vi "Begin.vi"(10 "Control Type":i8, 11 "Image Size":T1=enum."160x120") -> (0 "error out":errorcluster)   [LabVIEW 2011]
doc: "Called before other user functions, this VI is expected to open initial I/O refnums, load in file data, and do all program initialization. Notice that the <B>error out</B> terminal is simply used for data flow. Wiring it to other structures or subVIs ensures that this VI runs first."
uses:
  <vilib>/Rock Robotics/WPI/Camera/WPI_CameraImageSize.ctl
  <vilib>/Rock Robotics/WPI/Camera/WPI_CameraWhite Balance Values.ctl
  <vilib>/Rock Robotics/WPI/Camera/WPI_CameraExposure Values.ctl
  <vilib>/Rock Robotics/WPI/Camera/WPI_CameraFrameRate.ctl
  <vilib>/Rock Robotics/SystemInterfaces/Typedef/FPGA_TypedefAnalogModuleForGyro.ctl
  <vilib>/Rock Robotics/SystemInterfaces/AI/FPGA_AIGyroChannel.ctl
  <vilib>/Rock Robotics/SystemInterfaces/DIO/FPGA_DIOPWMChannel.ctl
  <vilib>/Rock Robotics/SystemInterfaces/Typedef/FPGA_TypedefDigitalModule.ctl
  <vilib>/Rock Robotics/SystemInterfaces/DIO/FPGA_DIOChannel.ctl
  <vilib>/Rock Robotics/SystemInterfaces/Typedef/FPGA_TypedefAnalogModule.ctl
  <vilib>/Rock Robotics/SystemInterfaces/AI/FPGA_AIChannel.ctl
  <vilib>/Rock Robotics/WPI/Encoder/WPI_EncoderType.ctl
  <vilib>/Rock Robotics/WPI/Joystick/WPI_JoystickDeviceEnum.ctl
  <vilib>/Rock Robotics/WPI/MotorControl/WPI_MotorControlOpen Victor.vi
  <vilib>/Rock Robotics/WPI/Counter/WPI_CounterDigitalInputToDigitalSource.vi
  <vilib>/Rock Robotics/WPI/RobotDrive/WPI_RobotDriveOpen4MotorWithVictor.vi
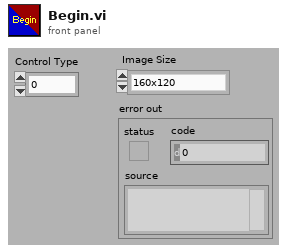
[diagram p1: front panel]
types:
  T1 = typedef "WPI_CameraImageSize.ctl" = enum16{"640x480", "320x240", "160x120"}
  T2 = typedef "WPI_EncoderType.ctl" = enum16{"1x", "2x", "4x"}
  T3 = typedef "FPGA_DIOChannel.ctl" = enum8{"DIO 1", "DIO 2", "DIO 3", "DIO 4", "DIO 5", "DIO 6", "DIO 7", "DIO 8", "DIO 9", "DIO 10", "DIO 11", "DIO 12", "DIO 13", "DIO 14", "Invalid"}
  T4 = typedef "FPGA_TypedefDigitalModule.ctl" = enum16{"Digital Module 1", "Digital Module 2"}
  T5 = typedef "FPGA_AIChannel.ctl" = enum8{"AI 1", "AI 2", "AI 3", "AI 4", "AI 5", "AI 6", "AI 7", "AI 8", "Invalid"}
  T6 = typedef "FPGA_TypedefAnalogModule.ctl" = enum16{"Analog Module 1", "Analog Module 2"}
  T7 = typedef "FPGA_DIOPWMChannel.ctl" = enum8{"PWM 1", "PWM 2", "PWM 3", "PWM 4", "PWM 5", "PWM 6", "PWM 7", "PWM 8", "PWM 9", "PWM 10", "Invalid"}
  T8 = typedef "FPGA_AIGyroChannel.ctl" = enum8{"AI 1", "AI 2", "Invalid"}
  T9 = typedef "FPGA_TypedefAnalogModuleForGyro.ctl" = enum16{"Analog Module 1"}
  T10 = typedef "WPI_CameraFrameRate.ctl" = u32
  T11 = typedef "WPI_CameraExposure Values.ctl" = enum16{"Auto", "Flicker-free 50 Hz", "Flicker-free 60 Hz", "Hold current"}
  T12 = typedef "WPI_CameraWhite Balance Values.ctl" = enum16{"Auto", "Fixed indoor", "Fixed outdoor 1", "Fixed outdoor 2", "Fixed fluorescent 1", "Fixed fluorescent 2", "Hold current"}
  T13 = typedef "WPI_MotorControlDeviceRef.ctl" = cluster{"DeviceStatus":errorcluster, "Type":enum16{"PWM", "CAN"}, "PWM":cluster{"Digital Module":T4, "PWM Channel":T7, "DeadBand":T14}, "CAN":cluster{"Device Number":u8, "Control Mode":T15, "Semaphore":T16, "Max Vout":dbl}, "Invert":bool, "TransformRef":T17, "InvTransformRef":T17}
  T14 = typedef "WPI_PWMDeadband.ctl" = cluster{"Name":string, "maxPositivePwm":i32, "minPositivePwm":i32, "centerPwm":i32, "maxNegativePwm":i32, "minNegativePwm":i32, "angularRange":u16}
  T15 = typedef "WPI_CANJaguar_ControlMode.ctl" = enum8{"Percent VBus", "Current", "Speed", "Position", "Voltage"}
  T16 = typedef "Semaphore RefNum" = refnum<k1>
  T17 = typedef "WPI_PWMTransform_ConPane.ctl" = refnum<vi>
  T18 = typedef "WPI_CameraDevRef.ctl" = cluster{"Camera Address":string, "CameraStatus":errorcluster, "Acquire Image Notifier":refnum<notifier>}
  T19 = typedef "WPI_RobotDriveDevRef.ctl" = cluster{"DevStatus":errorcluster, "Motors[]":T13[], "Square Inputs":bool, "Max Output":dbl, "Isochronous":bool}
  T20 = typedef "WPI_DigitalInputDevRef.ctl" = cluster{"DevStatus":errorcluster, "DIO Channel":T3, "Digital Module":T4}
  T21 = typedef "WPI_AnalogChannelDevRef.ctl" = cluster{"DevStatus":errorcluster, "Analog Module":T6, "Analog Channel":T5}
  T22 = typedef "WPI_GyroDevRef.ctl" = cluster{"DevStatus":errorcluster, "Analog Module":T6, "Analog Channel":T5, "Offset":dbl, "Gain (VoltsPerDegree/Second)":dbl}
  T23 = typedef "FPGA_CounterEncoderSourceConvertionLVSourceType.ctl" = cluster{"DevStatus":errorcluster, "AnalogTriggerMode?":bool, "DigitalMode":cluster{"Digital Module":T4, "DIO Channel":T24}, "AnalogTriggerMode":cluster{"AnalogTriggerIndex":T25, "OutputType":T26}}
  T24 = typedef "FPGA_DIODigitalSourceChannel.ctl" = enum8{"DIO 1", "DIO 2", "DIO 3", "DIO 4", "DIO 5", "DIO 6", "DIO 7", "DIO 8", "DIO 9", "DIO 10", "DIO 11", "DIO 12", "DIO 13", "DIO 14", "Disabled"}
  T25 = typedef "FPGA_AnalogTriggerIndex.ctl" = enum8{"Trig 0", "Trig 1", "Trig 2", "Trig 3", "Trig 4", "Trig 5", "Trig 6", "Trig 7", "Invalid"}
  T26 = typedef "FPGA_AnalogTriggerOutType.ctl" = enum16{"InWindow", "TriggerState", "Rising", "Falling"}
  T27 = typedef "WPI_EncoderDevRef.ctl" = cluster{"DevStatus":errorcluster, "EncoderIndex":T28, "CounterIndex":T29, "DistancePerCount":dbl, "Decoding Type":T2}
  T28 = typedef "FPGA_EncoderIdx.ctl" = enum8{"Enc 0", "Enc 1", "Enc 2", "Enc 3", "Invalid"}
  T29 = typedef "FPGA_CounterCtrSystemIndex.ctl" = enum8{"Ctr 0", "Ctr 1", "Ctr 2", "Ctr 3", "Ctr 4", "Ctr 5", "Ctr 6", "Ctr 7", "Invalid"}
  T30 = typedef "WPI_JoystickDeviceEnum.ctl" = enum16{"USB 1", "USB 2", "USB 3", "USB 4", "Kinect 1", "Kinect 2"}
  T31 = typedef "WPI_JoystickDevRef.ctl" = cluster{"Device":T30}
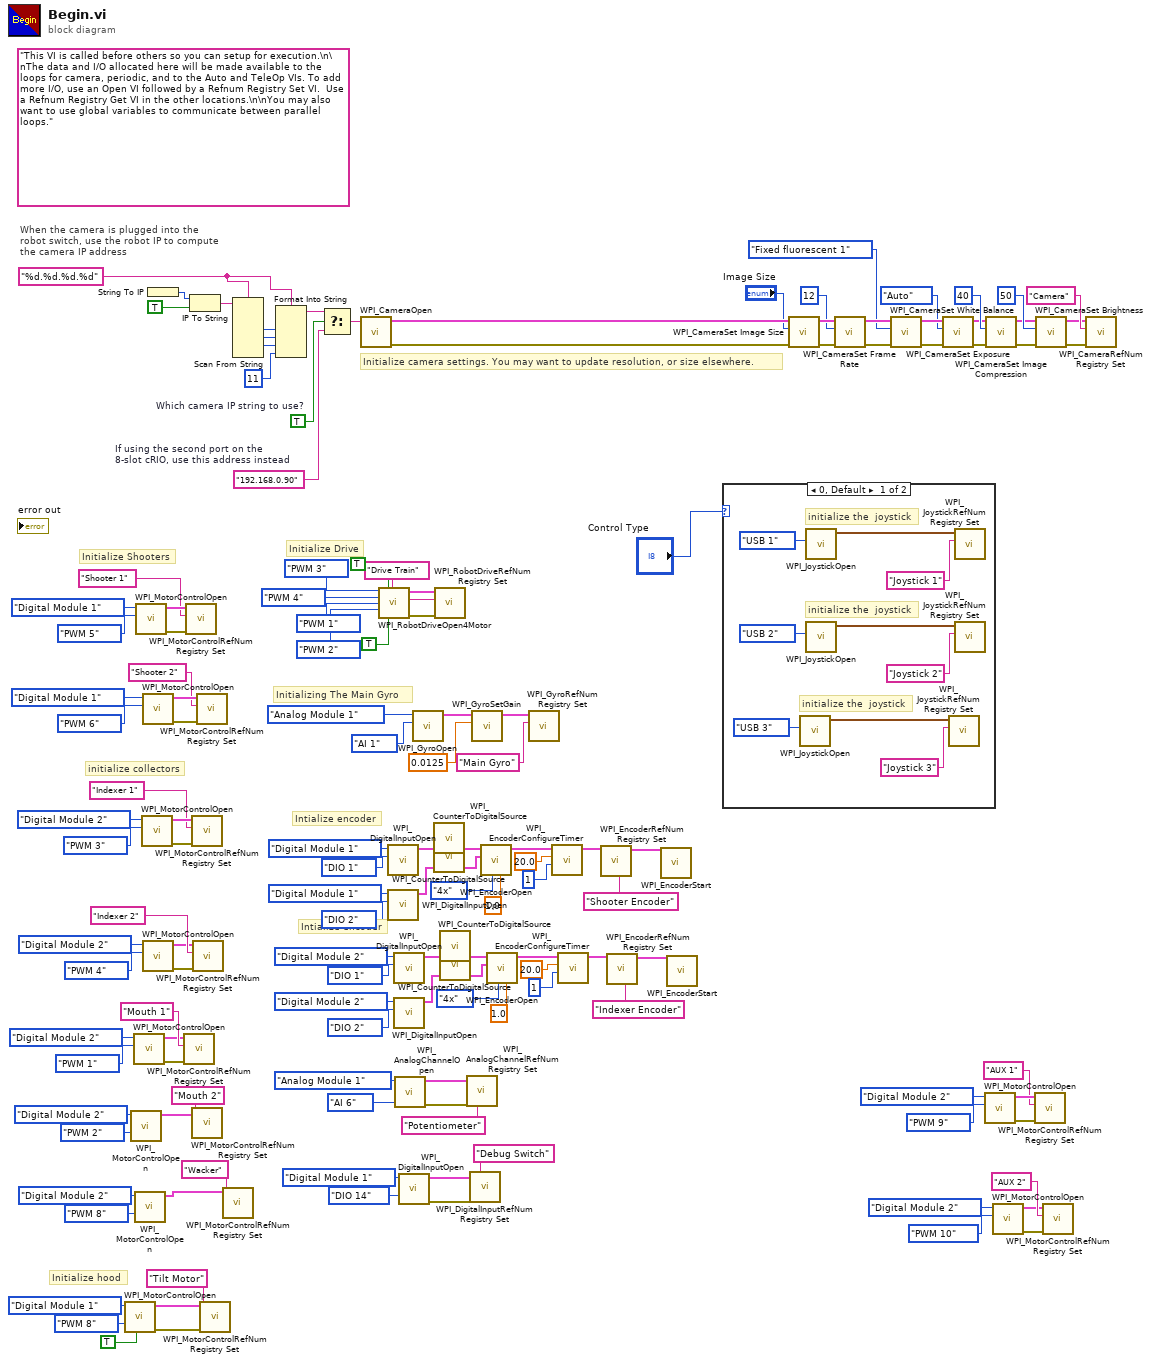
[diagram p0: block diagram]
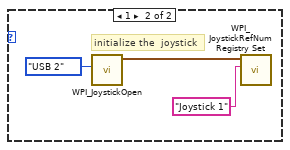
[diagram p2: hidden frame]
diagram:
  w108 = TRUE  # Which camera IP string to use?
  w112 = "%d.%d.%d.%d" ("format string")
  (unwired) "This VI is called before others so you can setup for execution.\n\nThe data and I/O allocated here will be made available to the loops for camera, periodic, and to the Auto and TeleOp VIs. To add more I/O, use an Open VI followed by a Refnum Registry Set VI.  Use a Refnum Registry Get VI in the other locations.\n\nYou may also want to use global variables to communicate between parallel loops."
  w109 = "192.168.0.90"  # If using the second port on the 8-slot cRIO, use this address instead
  # "Intialize encoder"
  # "Initialize hood"
  # "Intialize encoder"
  # "initialize collectors"
  # "Initialize Drive"
  # "Initializing The Main Gyro"
  # "Initialize Shooters"
  # "When the camera is plugged into the\nrobot switch, use the robot IP to compute\nthe camera IP address"
  # "Initialize camera settings. You may want to update resolution, or size elsewhere."
  n1 = call-poly <vilib>:"WPI_MotorControlOpen.vi"("Invert"=TRUE, "PWM Channel"=FPGA_DIOPWMChannel."PWM 8", "Digital Module (Module 1)"=FPGA_TypedefDigitalModule."Digital Module 1") -> ("error out"=w54:errorcluster, "MotorControlDeviceRef"=w58:T13)  [unwired: 7 in]
  n2 = call-poly <vilib>:"WPI_MotorControlOpen.vi"("PWM Channel"=FPGA_DIOPWMChannel."PWM 2", "Digital Module (Module 1)"=FPGA_TypedefDigitalModule."Digital Module 2") -> ("MotorControlDeviceRef"=w53:T13)  [unwired: 8 in, 1 out]
  n3 = call-poly <vilib>:"WPI_MotorControlOpen.vi"("PWM Channel"=FPGA_DIOPWMChannel."PWM 1", "Digital Module (Module 1)"=FPGA_TypedefDigitalModule."Digital Module 2") -> ("error out"=w81:errorcluster, "MotorControlDeviceRef"=w79:T13)  [unwired: 8 in]
  n4 = call-poly <vilib>:"WPI_MotorControlOpen.vi"("PWM Channel"=FPGA_DIOPWMChannel."PWM 8", "Digital Module (Module 1)"=FPGA_TypedefDigitalModule."Digital Module 2") -> ("MotorControlDeviceRef"=w49:T13)  [unwired: 8 in, 1 out]
  n5 = call-poly <vilib>:"WPI_MotorControlOpen.vi"("PWM Channel"=FPGA_DIOPWMChannel."PWM 5", "Digital Module (Module 1)"=FPGA_TypedefDigitalModule."Digital Module 1") -> ("error out"=w83:errorcluster, "MotorControlDeviceRef"=w87:T13)  [unwired: 8 in]
  n6 = call-poly <vilib>:"WPI_MotorControlOpen.vi"("PWM Channel"=FPGA_DIOPWMChannel."PWM 3", "Digital Module (Module 1)"=FPGA_TypedefDigitalModule."Digital Module 2") -> ("error out"=w92:errorcluster, "MotorControlDeviceRef"=w94:T13)  [unwired: 8 in]
  n7 = call-poly <vilib>:"WPI_MotorControlOpen.vi"("PWM Channel"=FPGA_DIOPWMChannel."PWM 6", "Digital Module (Module 1)"=FPGA_TypedefDigitalModule."Digital Module 1") -> ("error out"=w82:errorcluster, "MotorControlDeviceRef"=w86:T13)  [unwired: 8 in]
  n8 = call-poly <vilib>:"WPI_MotorControlOpen.vi"("PWM Channel"=FPGA_DIOPWMChannel."PWM 4", "Digital Module (Module 1)"=FPGA_TypedefDigitalModule."Digital Module 2") -> ("error out"=w47:errorcluster, "MotorControlDeviceRef"=w45:T13)  [unwired: 8 in]
  n9 = String To IP() -> (0:w119:u32)  [unwired: 1 in]
  n10 = call <vilib>:"WPI_MotorControlRefNum Registry Set.vi"("error in (no error)"=w81, "refnum name"="Mouth 1", "MotorControlDevRef"=w79) -> ()  [unwired: 7 in, 2 out]
  n11 = call <vilib>:"WPI_MotorControlRefNum Registry Set.vi"("error in (no error)"=w83, "refnum name"="Shooter 1", "MotorControlDevRef"=w87) -> ()  [unwired: 7 in, 2 out]
  n12 = IP To String(1:TRUE ("dot notation? (F)"), 2:w119) -> (0:w117:string)
  n13 = call <vilib>:"WPI_MotorControlRefNum Registry Set.vi"("error in (no error)"=w92, "refnum name"="Indexer 1", "MotorControlDevRef"=w94) -> ()  [unwired: 7 in, 2 out]
  n14 = call <vilib>:"WPI_MotorControlRefNum Registry Set.vi"("refnum name"="Mouth 2", "MotorControlDevRef"=w53) -> ()  [unwired: 8 in, 2 out]
  n15 = call <vilib>:"WPI_MotorControlRefNum Registry Set.vi"("error in (no error)"=w47, "refnum name"="Indexer 2", "MotorControlDevRef"=w45) -> ()  [unwired: 7 in, 2 out]
  n16 = call <vilib>:"WPI_MotorControlRefNum Registry Set.vi"("error in (no error)"=w82, "refnum name"="Shooter 2", "MotorControlDevRef"=w86) -> ()  [unwired: 7 in, 2 out]
  n17 = call <vilib>:"WPI_MotorControlRefNum Registry Set.vi"("error in (no error)"=w54, "refnum name"="Tilt Motor", "MotorControlDevRef"=w58) -> ()  [unwired: 7 in, 2 out]
  n18 = call <vilib>:"WPI_MotorControlRefNum Registry Set.vi"("refnum name"="Wacker", "MotorControlDevRef"=w49) -> ()  [unwired: 8 in, 2 out]
  n19 = Scan From String(format string=w112, input string=w117) -> (output 1=w116:i32, output 2=w115:i32, output 3=w114:i32)  [unwired: 7 in, 3 out]
  n20 = Format Into String(format string=w112, w116, w115, w114, 11 ("Compression")) -> (resulting string=w110:string)  [unwired: 2 in, 1 out]
  n21 = Select(t=w110, s=w108, f=w109) -> (s? t:f=w111:string)
  n22 = call <vilib>:"WPI_CameraOpen.vi"("Camera Address"=w111) -> ("error out"=w131:errorcluster, "CameraDevRef"=w132:T18)  [unwired: 1 in, 8 out]
  n23 = call-poly <vilib>:"WPI_RobotDriveOpen4Motor.vi"("Rear Left Motor"=FPGA_DIOPWMChannel."PWM 3", "Rear Left Motor Inverted"=TRUE, "Rear Right Motor"=FPGA_DIOPWMChannel."PWM 4", "Front Left Motor"=FPGA_DIOPWMChannel."PWM 1", "Front Right Motor"=FPGA_DIOPWMChannel."PWM 2", "Front Left Motor Inverted"=TRUE) -> ("RobotDriveDevRef"=w98:T19, "error out"=w97:errorcluster)  [unwired: 8 in]
  n24 = call <vilib>:"WPI_DigitalInputOpen.vi"("DIO Channel"=FPGA_DIOChannel."DIO 1", "Digital Module (Module 1)"=FPGA_TypedefDigitalModule."Digital Module 1") -> ("DigitalInputDevRef"=w74:T20)  [unwired: 8 in, 1 out]
  n25 = call <vilib>:"WPI_DigitalInputOpen.vi"("DIO Channel"=FPGA_DIOChannel."DIO 2", "Digital Module (Module 1)"=FPGA_TypedefDigitalModule."Digital Module 1") -> ("DigitalInputDevRef"=w70:T20)  [unwired: 8 in, 1 out]
  n26 = call <vilib>:"WPI_DigitalInputOpen.vi"("DIO Channel"=FPGA_DIOChannel."DIO 1", "Digital Module (Module 1)"=FPGA_TypedefDigitalModule."Digital Module 2") -> ("DigitalInputDevRef"=w14:T20)  [unwired: 8 in, 1 out]
  n27 = call <vilib>:"WPI_DigitalInputOpen.vi"("DIO Channel"=FPGA_DIOChannel."DIO 2", "Digital Module (Module 1)"=FPGA_TypedefDigitalModule."Digital Module 2") -> ("DigitalInputDevRef"=w10:T20)  [unwired: 8 in, 1 out]
  n28 = call <vilib>:"WPI_AnalogChannelOpen.vi"("Analog Channel"=FPGA_AIChannel."AI 6", "Analog Module (Module 1)"=FPGA_TypedefAnalogModule."Analog Module 1") -> ("error out"=w19:errorcluster, "AIDeviceRef"=w21:T21)  [unwired: 8 in]
  n29 = call <vilib>:"WPI_DigitalInputOpen.vi"("DIO Channel"=FPGA_DIOChannel."DIO 14", "Digital Module (Module 1)"=FPGA_TypedefDigitalModule."Digital Module 1") -> ("error out"=w24:errorcluster, "DigitalInputDevRef"=w26:T20)  [unwired: 8 in]
  n30 = call <vilib>:"WPI_GyroOpen.vi"("Analog Channel"=FPGA_AIGyroChannel."AI 1", "Analog Module (Module 1)"=FPGA_TypedefAnalogModuleForGyro."Analog Module 1") -> ("GyroDevRef"=w105:T22)  [unwired: 7 in, 2 out]
  n31 = call-poly <vilib>:"WPI_CounterToDigitalSource.vi"("DigitalInputDevRef"=w74) -> ("Digital Source"=w73:T23)  [unwired: 6 in]
  n32 = call-poly <vilib>:"WPI_CounterToDigitalSource.vi"("DigitalInputDevRef"=w70) -> ("Digital Source"=w69:T23)  [unwired: 6 in]
  n33 = call <vilib>:"WPI_RobotDriveRefNum Registry Set.vi"("error in (no error)"=w97, "refnum name"="Drive Train", "RobotDriveDevRef"=w98) -> ()  [unwired: 7 in, 2 out]
  n34 = call-poly <vilib>:"WPI_CounterToDigitalSource.vi"("DigitalInputDevRef"=w14) -> ("Digital Source"=w13:T23)  [unwired: 6 in]
  n35 = call-poly <vilib>:"WPI_CounterToDigitalSource.vi"("DigitalInputDevRef"=w10) -> ("Digital Source"=w9:T23)  [unwired: 6 in]
  n36 = call <vilib>:"WPI_AnalogChannelRefNum Registry Set.vi"("error in (no error)"=w19, "refnum name"="Potentiometer", "AIDeviceRef"=w21) -> ()  [unwired: 7 in, 2 out]
  n37 = call <vilib>:"WPI_DigitalInputRefNum Registry Set.vi"("error in (no error)"=w24, "refnum name"="Debug Switch", "DigitalInputDevRef"=w26) -> ()  [unwired: 7 in, 2 out]
  n38 = call <vilib>:"WPI_GyroSetGain.vi"("Gain (VoltsPerDegree/Second)"=0.0125, "GyroDevRef"=w105) -> ("GyroDevRef"=w103:T22)  [unwired: 8 in, 1 out]
  n39 = call <vilib>:"WPI_EncoderOpen.vi"("DistancePerCount"=1.0, "Decoding Type"=WPI_EncoderType."4x", "BSource"=w69, "ASource"=w73) -> ("EncoderDevRef"=w67:T27)  [unwired: 6 in, 1 out]
  n40 = call <vilib>:"WPI_EncoderOpen.vi"("DistancePerCount"=1.0, "Decoding Type"=WPI_EncoderType."4x", "BSource"=w9, "ASource"=w13) -> ("EncoderDevRef"=w7:T27)  [unwired: 6 in, 1 out]
  n41 = call <vilib>:"WPI_GyroRefNum Registry Set.vi"("refnum name"="Main Gyro", "GyroDevRef"=w103) -> ()  [unwired: 8 in, 2 out]
  n42 = call <vilib>:"WPI_EncoderConfigureTimer.vi"("Number Samples to Average"=u8 1, "Minimum Rate"=20.0, "EncoderDevRef"=w67) -> ("EncoderDevRef"=w65:T27)  [unwired: 7 in, 1 out]
  n43 = call <vilib>:"WPI_EncoderConfigureTimer.vi"("Number Samples to Average"=u8 1, "Minimum Rate"=20.0, "EncoderDevRef"=w7) -> ("EncoderDevRef"=w5:T27)  [unwired: 7 in, 1 out]
  n44 = call <vilib>:"WPI_EncoderRefNum Registry Set.vi"("refnum name"="Shooter Encoder", "EncoderDevRef"=w65) -> ("EncoderDevRef"=w18:T27)  [unwired: 8 in, 1 out]
  n45 = call <vilib>:"WPI_EncoderRefNum Registry Set.vi"("refnum name"="Indexer Encoder", "EncoderDevRef"=w5) -> ("EncoderDevRef"=w1:T27)  [unwired: 8 in, 1 out]
  n46 = call <vilib>:"WPI_EncoderStart.vi"("EncoderDevRef"=w18) -> ()  [unwired: 9 in, 2 out]
  n47 = call <vilib>:"WPI_EncoderStart.vi"("EncoderDevRef"=w1) -> ()  [unwired: 9 in, 2 out]
  n48 = case shown="0, Default" "Control Type" {
    frame 0, Default {
      # "initialize the  joystick"
      # "initialize the  joystick"
      # "initialize the  joystick"
      n49 = call <vilib>:"WPI_JoystickOpen.vi"("JoystickDevice"=WPI_JoystickDeviceEnum."USB 3") -> ("JoystickDevRef"=w143:T31)  [unwired: 10 out]
      n50 = call <vilib>:"WPI_JoystickOpen.vi"("JoystickDevice"=WPI_JoystickDeviceEnum."USB 1") -> ("JoystickDevRef"=w147:T31)  [unwired: 10 out]
      n51 = call <vilib>:"WPI_JoystickOpen.vi"("JoystickDevice"=WPI_JoystickDeviceEnum."USB 2") -> ("JoystickDevRef"=w144:T31)  [unwired: 10 out]
      n52 = call <vilib>:"WPI_JoystickRefNum Registry Set.vi"("refnum name"="Joystick 3", "JoystickDevRef"=w143) -> ()  [unwired: 1 in, 9 out]
      n53 = call <vilib>:"WPI_JoystickRefNum Registry Set.vi"("refnum name"="Joystick 1", "JoystickDevRef"=w147) -> ()  [unwired: 1 in, 9 out]
      n54 = call <vilib>:"WPI_JoystickRefNum Registry Set.vi"("refnum name"="Joystick 2", "JoystickDevRef"=w144) -> ()  [unwired: 1 in, 9 out]
    }
    frame 1 {
      # "initialize the  joystick"
      n55 = call <vilib>:"WPI_JoystickOpen.vi"("JoystickDevice"=WPI_JoystickDeviceEnum."USB 2") -> ("JoystickDevRef"=w150:T31)  [unwired: 10 out]
      n56 = call <vilib>:"WPI_JoystickRefNum Registry Set.vi"("refnum name"="Joystick 1", "JoystickDevRef"=w150) -> ()  [unwired: 1 in, 9 out]
    }
  }
  n57 = call <vilib>:"WPI_CameraSet Image Size.vi"("error in (no error)"=w131, "Image Size"="Image Size", "CameraDevRef"=w132) -> ("error out"=w130:errorcluster, "CameraDevRef Out"=w133:T18)  [unwired: 7 out]
  n58 = call <vilib>:"WPI_CameraSet Frame Rate.vi"("error in (no error)"=w130, "Frame Rate (fps)"=T10 12, "CameraDevRef"=w133) -> ("error out"=w129:errorcluster, "CameraDevRef Out"=w135:T18)  [unwired: 7 out]
  n59 = call <vilib>:"WPI_CameraSet White Balance.vi"("error in (no error)"=w129, "White Balance"=WPI_CameraWhite_Balance_Values."Fixed fluorescent 1", "CameraDevRef"=w135) -> ("error out"=w128:errorcluster, "CameraDevRef Out"=w134:T18)  [unwired: 7 out]
  n60 = call <vilib>:"WPI_CameraSet Exposure.vi"("error in (no error)"=w128, "Exposure"=WPI_CameraExposure_Values."Auto", "CameraDevRef"=w134) -> ("error out"=w127:errorcluster, "CameraDevRef Out"=w137:T18)  [unwired: 7 out]
  n61 = call-poly <vilib>:"WPI_MotorControlOpen.vi"("PWM Channel"=FPGA_DIOPWMChannel."PWM 9", "Digital Module (Module 1)"=FPGA_TypedefDigitalModule."Digital Module 2") -> ("error out"=w38:errorcluster, "MotorControlDeviceRef"=w40:T13)  [unwired: 8 in]
  n62 = call <vilib>:"WPI_CameraSet Image Compression.vi"("error in (no error)"=w127, "Compression"=40, "CameraDevRef"=w137) -> ("error out"=w126:errorcluster, "CameraDevRef Out"=w136:T18)  [unwired: 7 out]
  n63 = call-poly <vilib>:"WPI_MotorControlOpen.vi"("PWM Channel"=FPGA_DIOPWMChannel."PWM 10", "Digital Module (Module 1)"=FPGA_TypedefDigitalModule."Digital Module 2") -> ("error out"=w37:errorcluster, "MotorControlDeviceRef"=w35:T13)  [unwired: 8 in]
  n64 = call <vilib>:"WPI_MotorControlRefNum Registry Set.vi"("error in (no error)"=w38, "refnum name"="AUX 1", "MotorControlDevRef"=w40) -> ()  [unwired: 7 in, 2 out]
  n65 = call <vilib>:"WPI_CameraSet Brightness.vi"("error in (no error)"=w126, "Brightness"=50, "CameraDevRef"=w136) -> ("error out"=w124:errorcluster, "CameraDevRef Out"=w125:T18)  [unwired: 7 out]
  n66 = call <vilib>:"WPI_MotorControlRefNum Registry Set.vi"("error in (no error)"=w37, "refnum name"="AUX 2", "MotorControlDevRef"=w35) -> ()  [unwired: 7 in, 2 out]
  n67 = call <vilib>:"WPI_CameraRefNum Registry Set.vi"("error in (no error)"=w124, "refnum name"="Camera", "CameraDevRef"=w125) -> ()  [unwired: 9 out]
